vi "_emi_SMLoop Get State Array.vi"(5 "Loop IDs":u16[](array[numeric]), 9 "error in (no error)":errorcluster) -> (1 "Any Enabled, not running, trice":bool, 2 "Any Enabled, not running, twice":bool, 3 "Any Enabled, not running":bool, 6 "Loop IDs out":u16[](array[numeric]), 8 "All Loop Running Out":bool, 10 "error out":errorcluster, 14 "All Loop Enable Out":bool)   [LabVIEW 2011]
doc: "Retreive the execution state of the loop designated by Index. Used to syncronice different loops in teh same master loop.\n\nTo discover if the loop is failing to start, or has stopped unnececerily, check if \"Enabled, not running, twice \" or Trice is True. (Once can easily detect delay between Enablke and start). Distance between calls needs to be greater then the SMLoops Standby time."
uses:
  Loop control/Private/_emi_Loop control int action.ctl
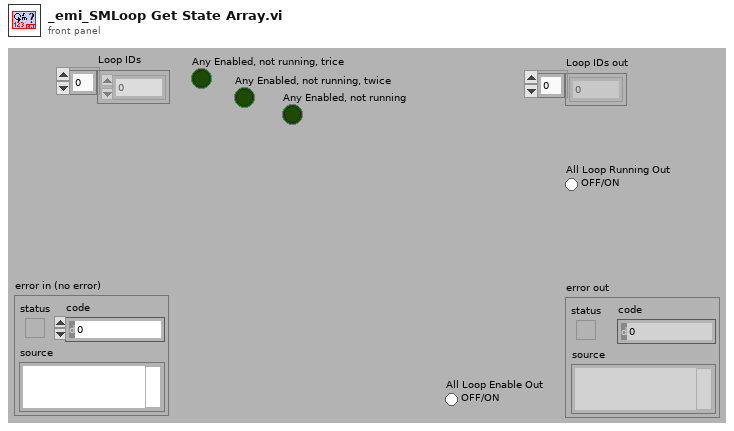
[diagram p1: front panel]
types:
  T1 = typedef "_emi_Loop control int action.ctl" = enum16{"Init index", "Get index", "Set index", "Get Size"}
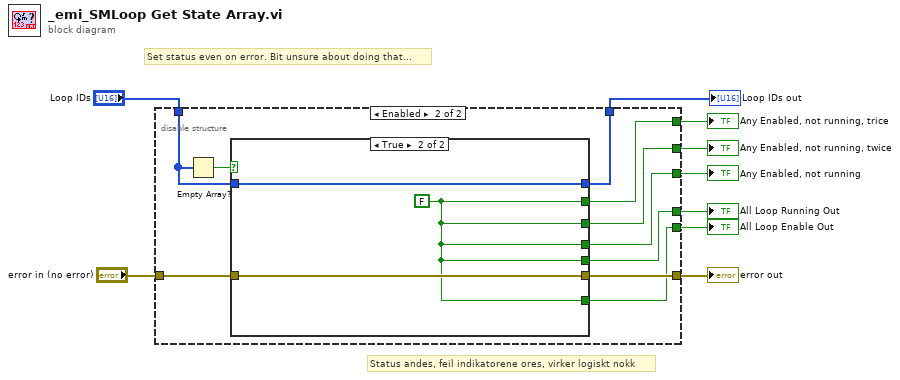
[diagram p0: block diagram]
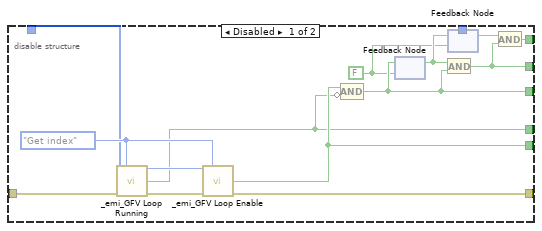
[diagram p2: hidden frame]
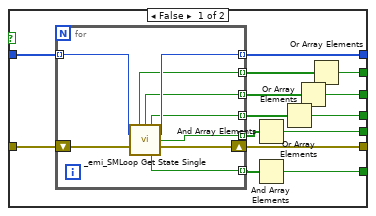
[diagram p3: hidden frame]
diagram:
  # "Status andes, feil indikatorene ores, virker logiskt nokk"
  # "Set status even on error. Bit unsure about doing that..."
  n1 = disable-structure shown="Enabled" {
    disable-tunnel: "error in (no error)" -> [w24 w32]
    disable-tunnel: [w22 w31] -> w8
    disable-tunnel: [w18 w25] -> w7
    disable-tunnel: [w17 w27] -> w6
    disable-tunnel: [w14 w28] -> w5
    disable-tunnel: [w13 w29] -> w4
    disable-tunnel: "Loop IDs" -> [w11 w33]
    disable-tunnel: [w10 w26] -> w2
    disable-tunnel: [_ w30] -> w1
    frame Disabled {
      w12 = FALSE
      w21 = _emi_Loop_control_int_action."Get index" ("Action(Get Index)")
      n2 = call "_emi_GFV Loop Running.vi"("Loop Index/Numb"=w11, "Action(Get Index)"=w21, "error in (no error)"=w24) -> ("Index out"=w20:u16, "Loop Running Out"=w10:bool, "error out"=w23:errorcluster)  [unwired: 9 in, 1 out]
      n3 = call "_emi_GFV Loop Enable.vi"("Loop Index/Numb"=w20, "Action(Get Index)"=w21, "error in (no error)"=w23) -> ("Index out"=w19:u16, "Loop Enable Out"=w18:bool, "error out"=w22:errorcluster)  [unwired: 9 in, 1 out]
      n4 = Compound Arithmetic op=AND(w18, invert w10) -> (w17:bool)
      n5 = feedback #1(w12) -> (w16:bool)
      n6 = feedback-in #1(w17) -> ()
      n7 = And(x=w16, y=w17) -> (x .and. y?=w14:bool)
      n8 = feedback #2(w12) -> (w15:bool)
      n9 = feedback-in #2(w16) -> ()
      n10 = And(x=w15, y=w14) -> (x .and. y?=w13:bool)
    }
    frame Enabled {
      n11 = Empty Array?(array=w33) -> (empty?=w34:bool)
      n12 = case shown="True" w34 {
        tunnel: w33 -> [w46 w59]
        tunnel: w32 -> [w48 w60]
        tunnel: [w47 w60] -> w31
        tunnel: [w45 w59] -> w30
        tunnel: [w43 w58] -> w25
        tunnel: [w41 w58] -> w26
        tunnel: [w37 w58] -> w29
        tunnel: [w36 w58] -> w28
        tunnel: [w35 w58] -> w27
        frame False {
          n13 = for {
            shift-right: [w56] -> w47
            shift-left: w48 -> [w57]
            tunnel: w46 -> [w55] mode=indexing
            tunnel: [w54] -> w45 mode=indexing
            tunnel: [w53] -> w44 mode=indexing
            tunnel: [w52] -> w42 mode=indexing
            tunnel: [w51] -> w40 mode=indexing
            tunnel: [w50] -> w39 mode=indexing
            tunnel: [w49] -> w38 mode=indexing
            n14 = call "_emi_SMLoop Get State Single.vi"("Loop ID in"=w55, "error in (no error)"=w57) -> ("Enabled, not running, trice"=w49:bool, "Enabled, not running, twice"=w50:bool, "Enabled, not running"=w51:bool, "Loop ID out"=w54:u16, "Loop Running Out"=w52:bool, "error out"=w56:errorcluster, "Loop Enable Out"=w53:bool)  [unwired: 7 in]
          }
          n15 = And Array Elements(Boolean array=w42) -> (logical AND=w41:bool)
          n16 = And Array Elements(Boolean array=w44) -> (logical AND=w43:bool)
          n17 = Or Array Elements(Boolean array=w40) -> (logical OR=w35:bool)
          n18 = Or Array Elements(Boolean array=w39) -> (logical OR=w36:bool)
          n19 = Or Array Elements(Boolean array=w38) -> (logical OR=w37:bool)
        }
        frame True {
          w58 = FALSE
        }
      }
    }
  }
  "error out" <- w8
  "All Loop Running Out" <- w2
  "All Loop Enable Out" <- w7
  "Any Enabled, not running" <- w6
  "Any Enabled, not running, twice" <- w5
  "Any Enabled, not running, trice" <- w4
  "Loop IDs out" <- w1
